vi "main.vi"   [LabVIEW 2015]
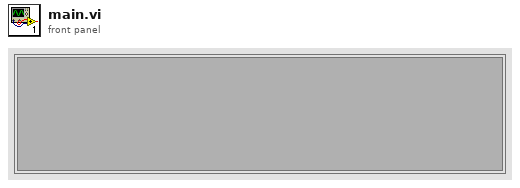
[diagram p1: front panel]
types:
  T1 = typedef "Window Refnum" = refnum<k1>
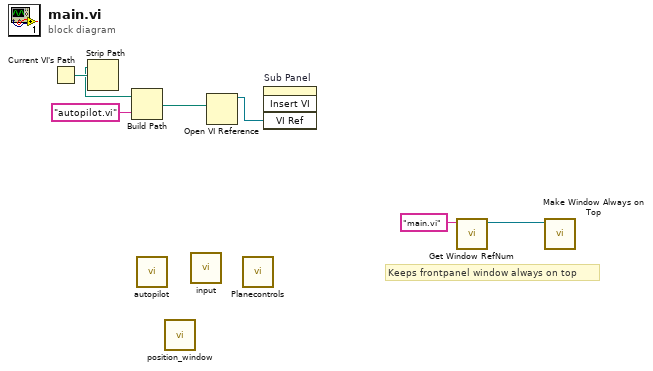
[diagram p0: block diagram]
diagram:
  # "Keeps frontpanel window always on top"
  n1 = Current VI's Path() -> (path=w7:path)
  n2 = Strip Path(path=w7) -> (stripped path=w6:path)  [unwired: 1 out]
  n3 = Build Path(base path=w6, name or relative path="autopilot.vi") -> (appended path=w4:path)
  n4 = call "autopilot.vi"() -> ()  [unwired: 12 in]
  n5 = call "position_window.vi"() -> ()  [unwired: 12 in]
  n6 = call "input.vi"() -> ()  [unwired: 12 in]
  n7 = Open VI Reference(vi path=w4) -> (vi reference=w3:refnum<vi>)  [unwired: 5 in, 1 out]
  n8 = call "Planecontrols.vi"() -> ()  [unwired: 12 in]
  n9 = invoke on="Sub Panel" class="SubPnl" method="Insert VI"("VI Ref"=w3) -> ()  [unwired: 3 in, 4 out]
  n10 = call "Get Window RefNum.vi"("window name (\"\")"="main.vi" ("window name (\"\")")) -> ("window refnum (NaWR)"=w1:T1)  [unwired: 7 in, 1 out]
  n11 = call "Make Window Always on Top.vi"("window refnum (NaWR)"=w1) -> ()  [unwired: 5 in, 2 out]
